vi "Calibrator.vi"(0 "data server address":string="dataserver.cee.cornell.edu", 2 "Channels":T17 items=["SC1Mod1/ai0", "SC1Mod1/ai1", "SC1Mod1/ai2", "SC1Mod1/ai3", "SC1Mod1/ai4", "SC1Mod1/ai5", "SC1Mod1/ai6", "SC1Mod1/ai7", "SC1Mod1/ai8", "SC1Mod1/ai9", "SC1Mod1/ai10", "SC1Mod1/ai11", "SC1Mod1/ai12", "SC1Mod1/ai13", "SC1Mod1/ai14", "SC1Mod1/ai15", "SC1Mod1/ai16", "SC1Mod1/ai17", "SC1Mod1/ai18", "SC1Mod1/ai19", "SC1Mod1/ai20", "SC1Mod1/ai21", "SC1Mod1/ai22", "SC1Mod1/ai23", "SC1Mod1/ai24", "SC1Mod1/ai25", "SC1Mod1/ai26", "SC1Mod1/ai27", "SC1Mod1/ai28", "SC1Mod1/ai29", "SC1Mod1/ai30", "SC1Mod1/ai31", "SC1Mod2/ai0", "SC1Mod2/ai1", "SC1Mod2/ai2", "SC1Mod2/ai3", "SC1Mod2/ai4", "SC1Mod2/ai5", "SC1Mod2/ai6", "SC1Mod2/ai7", "SC1Mod2/ai8", "SC1Mod2/ai9", "SC1Mod2/ai10", "SC1Mod2/ai11", "SC1Mod2/ai12", "SC1Mod2/ai13", "SC1Mod2/ai14", "SC1Mod2/ai15", "SC1Mod2/ai16", "SC1Mod2/ai17", "SC1Mod2/ai18", "SC1Mod2/ai19", "SC1Mod2/ai20", "SC1Mod2/ai21", "SC1Mod2/ai22", "SC1Mod2/ai23", "SC1Mod2/ai24", "SC1Mod2/ai25", "SC1Mod2/ai26", "SC1Mod2/ai27", "SC1Mod2/ai28", "SC1Mod2/ai29", "SC1Mod2/ai30", "SC1Mod2/ai31", "SC1Mod3/ai0", "SC1Mod3/ai1", "SC1Mod3/ai2", "SC1Mod3/ai3", "SC1Mod3/ai4", "SC1Mod3/ai5", "SC1Mod3/ai6", "SC1Mod3/ai7", "SC1Mod3/ai8", "SC1Mod3/ai9", "SC1Mod3/ai10", "SC1Mod3/ai11", "SC1Mod3/ai12", "SC1Mod3/ai13", "SC1Mod3/ai14", "SC1Mod3/ai15", "SC1Mod3/ai16", "SC1Mod3/ai17", "SC1Mod3/ai18", "SC1Mod3/ai19", "SC1Mod3/ai20", "SC1Mod3/ai21", "SC1Mod3/ai22", "SC1Mod3/ai23", "SC1Mod3/ai24", "SC1Mod3/ai25", "SC1Mod3/ai26", "SC1Mod3/ai27", "SC1Mod3/ai28", "SC1Mod3/ai29", "SC1Mod3/ai30", "SC1Mod3/ai31", "SC1Mod4/ai0", "SC1Mod4/ai1", "SC1Mod4/ai2", "SC1Mod4/ai3", "SC1Mod4/ai4", "SC1Mod4/ai5", "SC1Mod4/ai6", "SC1Mod4/ai7", "SC1Mod4/ai8", "SC1Mod4/ai9", "SC1Mod4/ai10", "SC1Mod4/ai11", "SC1Mod4/ai12", "SC1Mod4/ai13", "SC1Mod4/ai14", "SC1Mod4/ai15", "SC1Mod4/ai16", "SC1Mod4/ai17", "SC1Mod4/ai18", "SC1Mod4/ai19", "SC1Mod4/ai20", "SC1Mod4/ai21", "SC1Mod4/ai22", "SC1Mod4/ai23", "SC1Mod4/ai24", "SC1Mod4/ai25", "SC1Mod4/ai26", "SC1Mod4/ai27", "SC1Mod4/ai28", "SC1Mod4/ai29", "SC1Mod4/ai30", "SC1Mod4/ai31"]) -> (7 "sensor file path":path, 9 "Ports out":T17, 10 "Sensor Names":string[](array[string]))   [LabVIEW 2012]
uses:
  toolbar icons/Save configuration.ctl
  toolbar icons/Save calibration.ctl
  toolbar icons/open configuration.ctl
  toolbar icons/Open calibration.ctl
  toolbar icons/simultaneous standard cal.ctl
  toolbar icons/NF90 cal.ctl
  toolbar icons/pH cal.ctl
  toolbar icons/D.O. cal.ctl
  TCP DAQ/Set.ctl
  TCP DAQ/clear offset.ctl
  toolbar icons/Edit calibration.ctl
  toolbar icons/copy sensor.ctl
  toolbar icons/insert sensor.ctl
  toolbar icons/delete sensor.ctl
  DAQ configuration/Sensor array.ctl
  DAQ configuration/channel identifier.ctl
  calibrator graph.ctl
  toolbar icons/help.ctl
  TCP DAQ/Sensor data.ctl
  DAQ configuration/sensor cluster.ctl
  conversion.ctl
  DAQ configuration/scale type.ctl
  correspondence table.ctl
  pH/pH scale.ctl
  Dissolved Oxygen/DO scale.ctl
  calib array.ctl
  TCP DAQ/zero.ctl
  DAQ configuration/Sensor buffer command.ctl
  global scale array.vi
  DataServer/Server Stats.vi
panel:
  out "number of available channels":u16
  in  "Zero":T1
  in  "Sensor List":i32(listbox)=-1
  in  "Save configuration":T2
  in  "Save calibration":T3
  in  "Open configuration":T4
  in  "Open calibration":T5
  in  "units":string
  in  "name":string
  in  "Simultaneous Standard":T6
  in  "nf90":T7
  in  "pH":T8
  in  "DO":T9
  in  "Set clear":T12 {"target value" format="%.1p"}
  in  "Edit calibration":T13
  in  "Cancel":bool
  in  "Duplicate Sensor":T14
  in  "Add Sensor":T15
  in  "Delete Sensor":T16
  in  "OK":bool
  in  "data rate (ms)":u32=10
  in  "history length":u16=100 min=1
  out "Data Display":T19 {"average data rate (Hz)" format="%.2f"; "Min Range" format="%.3f"; "Max Range" format="%.3f"; "Mean (Volts)" format="%.5f"; "Mean (scaled)" format="%.2f"}
  out "Initial Calibration matrix":T20 {"D.O."."K" format="%.6f"; "D.O."."Temperature" format="%.2f"; "pH scale"."Buffers"."V/T" format="%.5f"; "pH scale"."Buffers"."Buffer" format="%.2f"; "pH scale"."Temperature" format="%.2f"; "offset (physical units)" format="%.5f"; "correspondence table"."volts" format="%.4f"; "correspondence table"."physical units" format="%.4f"; "second channel" min=-1; "offset (volts)" format="%.5f"; "conversion matrix" format="%.4e"}
  in  "Volts":T21={"conversion matrix"=[[0.0, 0.0], [0.0, 0.0], [0.0, 0.0], [0.0, 0.0], [0.0, 0.0], [0.0, 0.0]], "units"="volts", "name"="", "scale type"=enum."Volts", "offset (volts)"=0.0, "second channel"=0, "correspondence table"=[], "offset (physical units)"=0.0, "pH scale"={"Buffers"=[], "Temperature"=0.0}, "D.O."={"Temperature"=0.0, "K"=0.0, "barometric pressure"=0.0}} {"D.O."."K" format="%.6f"; "D.O."."Temperature" format="%.2f"; "pH scale"."Buffers"."V/T" format="%.5f"; "pH scale"."Buffers"."Buffer" format="%.2f"; "pH scale"."Temperature" format="%.2f"; "offset (physical units)" format="%.5f"; "correspondence table"."volts" format="%.4f"; "correspondence table"."physical units" format="%.4f"; "second channel" min=-1; "offset (volts)" format="%.5f"; "conversion matrix" format="%.4e"}
  out "Initial Ports":T17
  out "Sensor Data":T26 {"Sensor array"."scaled" format="%.2f"; "Sensor array"."voltage" format="%.4f"; "Time" format="%<%I:%M:%S%2u %p\n%m/%d/%Y>T"}
  in  "Help":T28
  in  "stop":bool
  # "V"
  # "V"
  # "C"
  # "kPa"
  # "C"
  # "C"
  # "kPa"
  # "C"
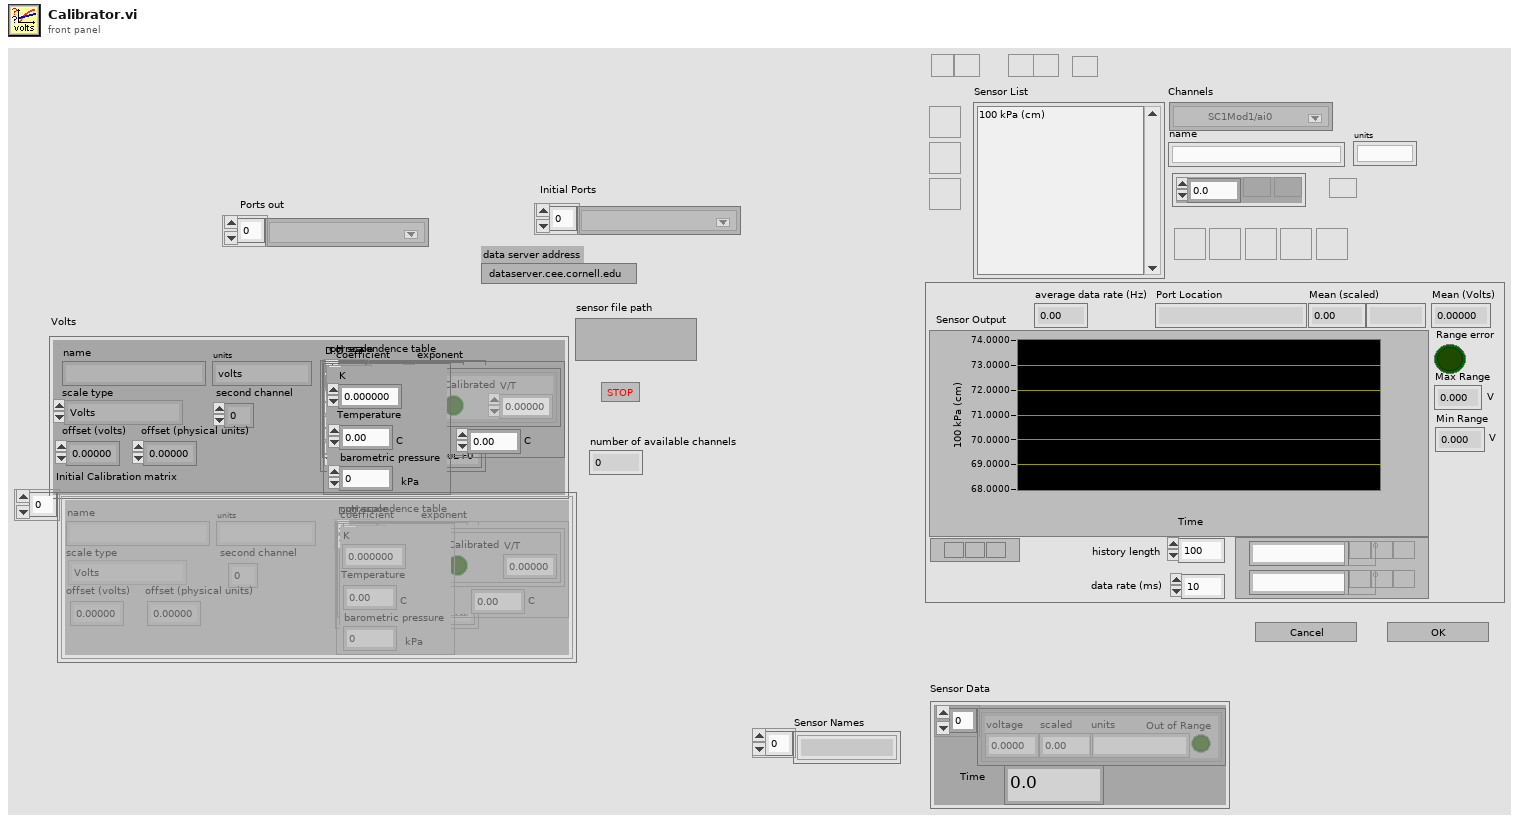
[diagram p1: front panel]
types:
  T1 = typedef "zero.ctl" = bool
  T2 = typedef "Save configuration.ctl" = bool
  T3 = typedef "Save calibration.ctl" = bool
  T4 = typedef "open configuration.ctl" = bool
  T5 = typedef "Open calibration.ctl" = bool
  T6 = typedef "simultaneous standard cal.ctl" = bool
  T7 = typedef "NF90 cal.ctl" = bool
  T8 = typedef "pH cal.ctl" = bool
  T9 = typedef "D.O. cal.ctl" = bool
  T10 = typedef "Set.ctl" = bool
  T11 = typedef "clear offset.ctl" = bool
  T12 = cluster{"Set":T10, "target value":dbl, "Clear":T11}
  T13 = typedef "Edit calibration.ctl" = bool
  T14 = typedef "copy sensor.ctl" = bool
  T15 = typedef "insert sensor.ctl" = bool
  T16 = typedef "delete sensor.ctl" = bool
  T17 = typedef "Sensor array.ctl" = T18[]
  T18 = typedef "channel identifier.ctl" = u16
  T19 = typedef "calibrator graph.ctl" = cluster{"Range error":bool, "Mean (scaled)":dbl, "Mean (Volts)":dbl, "Max Range":dbl, "Min Range":dbl, "units":string, "Sensor Output":cluster{dbl[], dbl[]}[], "Port Location":string, "average data rate (Hz)":dbl}
  T20 = typedef "calib array.ctl" = T21[]
  T21 = typedef "conversion.ctl" = cluster{"conversion matrix":sgl[][], "units":string, "name":string, "scale type":T22, "offset (volts)":dbl, "second channel":i8, "correspondence table":T23, "offset (physical units)":dbl, "pH scale":T24, "D.O.":T25}
  T22 = typedef "scale type.ctl" = enum16{"Volts", "Polynomial", "Correspondence Table", "pH", "Dissolved Oxygen", "Quadratic"}
  T23 = typedef "correspondence table.ctl" = cluster{"physical units":dbl, "volts":dbl}[]
  T24 = typedef "pH scale.ctl" = cluster{"Buffers":cluster{"Buffer":dbl, "Calibrated":bool, "V/T":dbl}[], "Temperature":dbl}
  T25 = typedef "DO scale.ctl" = cluster{"Temperature":dbl, "K":dbl, "barometric pressure":dbl}
  T26 = typedef "Sensor data.ctl" = cluster{" Sensor array":T27[], "Time":dbl}
  T27 = typedef "sensor cluster.ctl" = cluster{"voltage":sgl, "scaled":sgl, "units":string, "Out of Range":bool}
  T28 = typedef "help.ctl" = bool
  T29 = typedef "Sensor buffer command.ctl" = enum16{"read average", "read recent", "read all", "write", "configure", "clear"}
  T30 = typedef "Server stats.ctl" = cluster{"scan rate":dbl, "# connections":i32, "channel settings":cluster{"Name":string, "upper input limits":sgl, "lower input limits":sgl, "Location":string}[]}
  T31 = cluster{"Name":string, "upper input limits":sgl, "lower input limits":sgl, "Location":string}[]
  T32 = cluster{"Name":string, "upper input limits":sgl, "lower input limits":sgl, "Location":string}
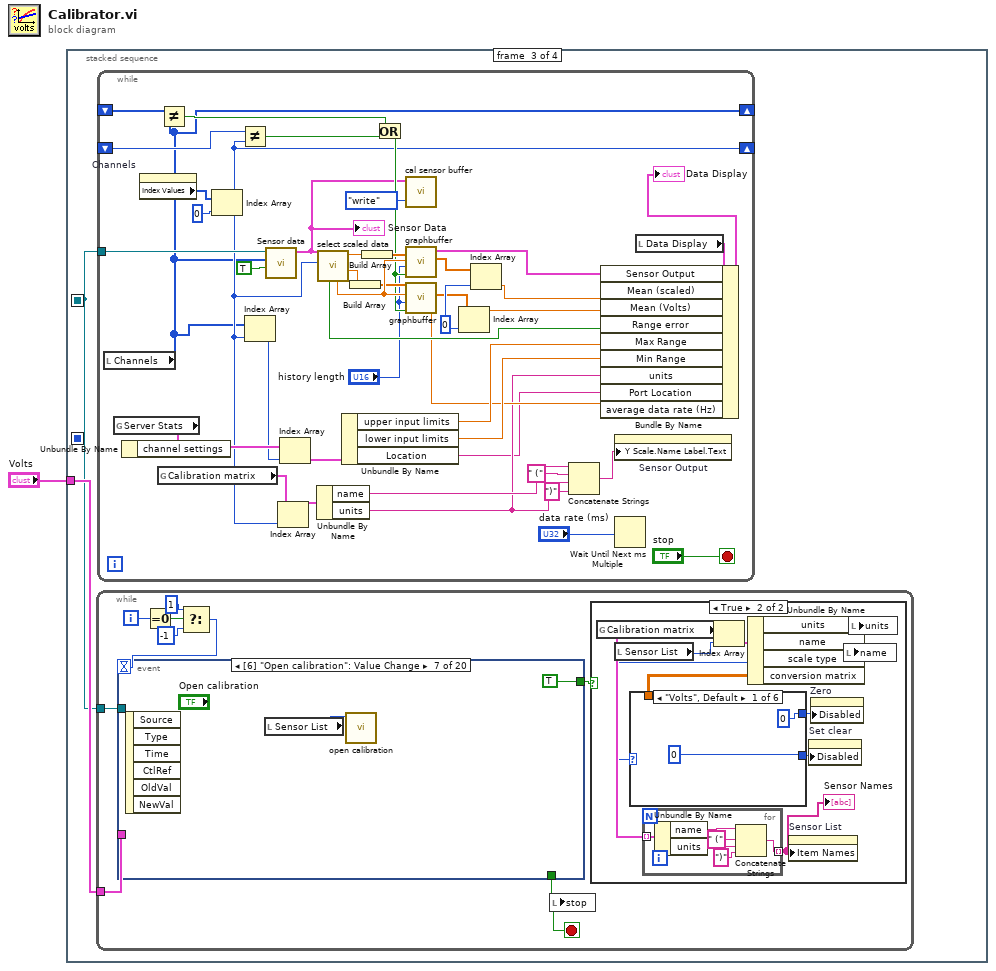
[diagram p0: block diagram]
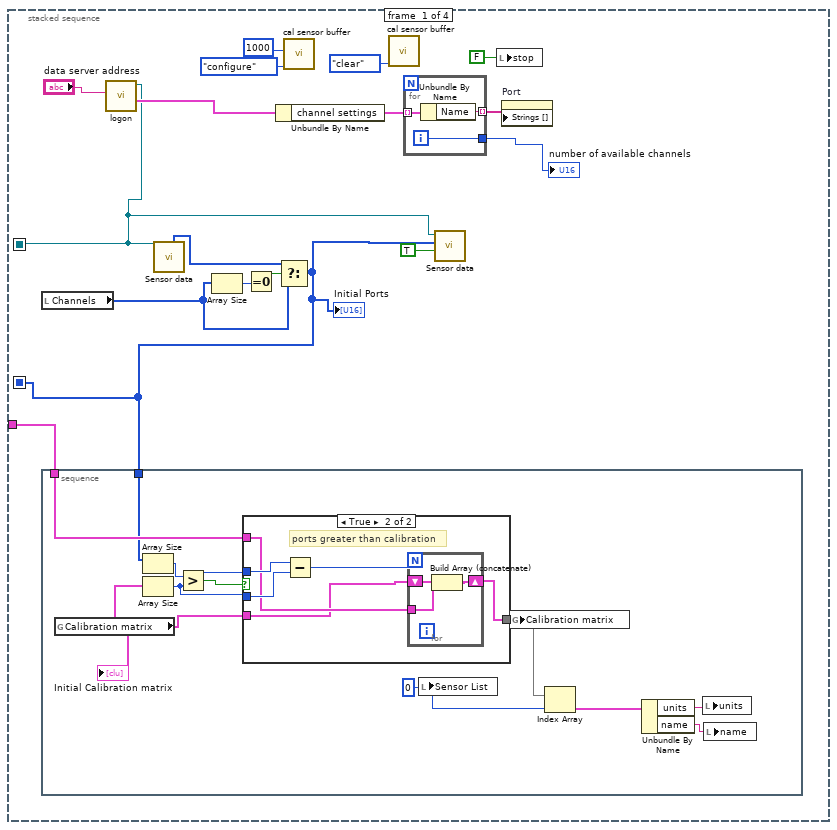
[diagram p2: hidden frame]
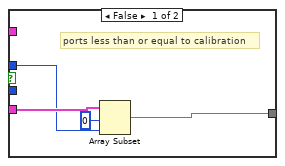
[diagram p3: hidden frame]
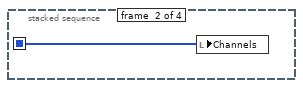
[diagram p4: hidden frame]
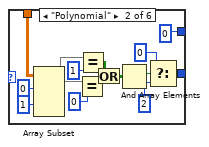
[diagram p6: hidden frame]
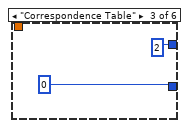
[diagram p7: hidden frame]
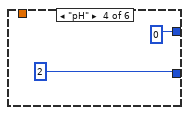
[diagram p8: hidden frame]
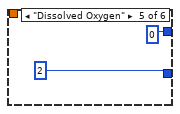
[diagram p9: hidden frame]
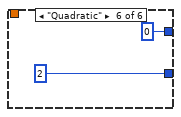
[diagram p10: hidden frame]
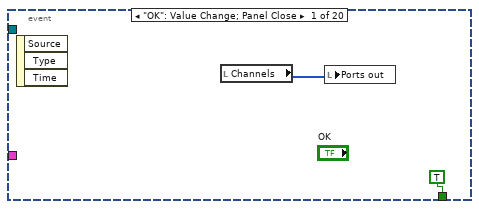
[diagram p11: hidden frame]
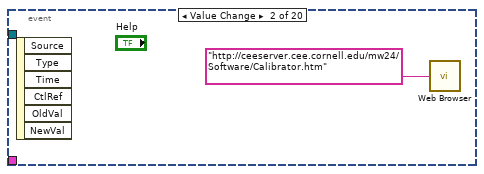
[diagram p12: hidden frame]
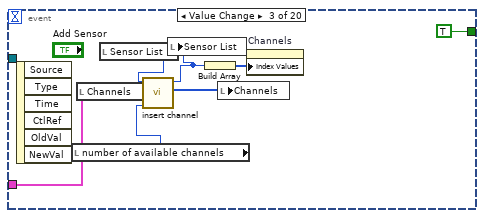
[diagram p13: hidden frame]
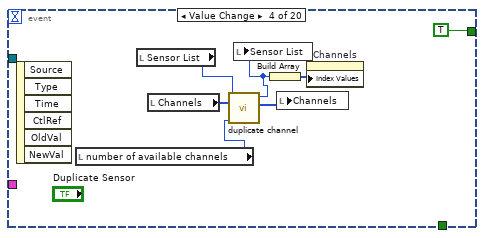
[diagram p14: hidden frame]
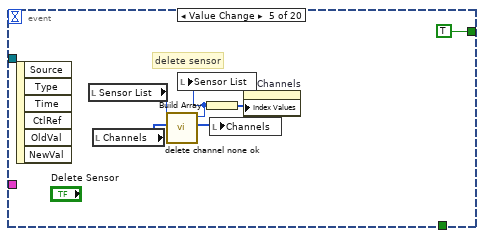
[diagram p15: hidden frame]
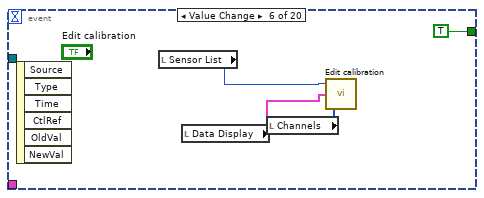
[diagram p16: hidden frame]
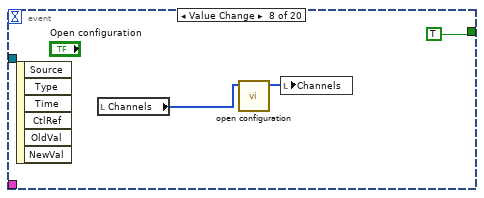
[diagram p17: hidden frame]
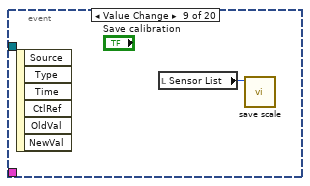
[diagram p18: hidden frame]
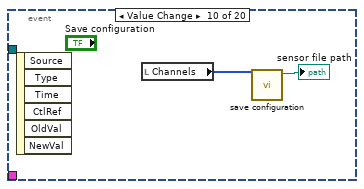
[diagram p19: hidden frame]
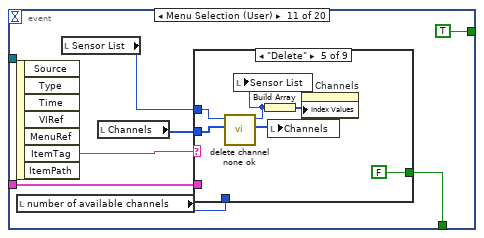
[diagram p20: hidden frame]
diagram:
  n1 = stacked-sequence {
    seq-local: [w6 _ _ _] -> [_ _ w47 w266]
    seq-local: [w2 _ _ _] -> [_ w46 _ _]
    tunnel: "Volts" -> [w18 _ w48 _]
    frame #0 {
      n2 = local read "Channels"() -> (w3:T17)
      n3 = call "logon.vi"("data server address in"="data server address") -> ("Server stats"=w9:T30, "connection ID"=w6:refnum<k5>)  [unwired: 7 in, 2 out]
      n4 = call "Sensor data.vi"("Connection ID in"=w6) -> ("Sensor Array out"=w12:T17)  [unwired: 3 in, 7 out]
      n5 = Array Size(array=w3) -> (size(s)=w11:i32)
      n6 = Equal To 0?(x=w11) -> (x = 0?=w10:bool)
      n7 = Unbundle By Name(w9) -> ("channel settings"=w8:T31)
      n8 = Select(t=w12, s=w10, f=w3) -> (s? t:f=w2:T17)
      "Initial Ports" <- w2
      n9 = stacked-sequence {
        tunnel: w18 -> [w28]
        tunnel: w2 -> [w22]
        frame #0 {
          w27 = u32 0 ("Index")
          n10 = global read "global scale array.vi" "Calibration matrix"() -> (w32:T20)
          "Initial Calibration matrix" <- w32
          n11 = Array Size(array=w22) -> (size(s)=w31:i32)
          n12 = Array Size(array=w32) -> (size(s)=w30:i32)
          n13 = Greater?(x=w31, y=w30) -> (0:w29:bool)
          n14 = case shown="True" w29 {
            tunnel: w31 -> [w35 w42]
            tunnel: w30 -> [_ w41]
            tunnel: w28 -> [_ w40]
            tunnel: w32 -> [w36 w37]
            tunnel: [w33 w38] -> w23
            frame False {
              # "ports less than or equal to calibration"
              n15 = Array Subset(array=w36, index=0 ("Array Index"), length=w35) -> (w33:T20)
            }
            frame True {
              # "ports greater than calibration"
              n16 = Subtract(x=w42, y=w41) -> (x-y=w39:i32)
              n17 = for {
                N: w39 -> [_]
                tunnel: w40 -> [w45]
                shift-right: [w43] -> w38
                shift-left: w37 -> [w44]
                n18 = Build Array (concatenate)(w44, w45) -> (w43:T20)
              }
            }
          }
          n19 = local write "Sensor List"(w27) -> ()
          n20 = global write "global scale array.vi" "Calibration matrix"(w23) -> ()
          n21 = Index Array(array=w23, index=w27) -> (element=w26:T21)
          n22 = Unbundle By Name(w26) -> ("units"=w25:string, "name"=w24:string)
          n23 = local write "units"(w25) -> ()
          n24 = local write "name"(w24) -> ()
        }
      }
      n25 = call "cal sensor buffer.vi"("command"=Sensor_buffer_command."configure", "max array size"=u16 1000) -> ()  [unwired: 3 in, 3 out]
      n26 = call "cal sensor buffer.vi"("command"=Sensor_buffer_command."clear") -> ()  [unwired: 4 in, 3 out]
      n27 = for {
        tunnel: w8 -> [w21] mode=indexing
        tunnel: [w20] -> w7 mode=indexing
        tunnel: [w19] -> w4
        i -> [w19]
        n28 = Unbundle By Name(w21) -> ("Name"=w20:string)
      }
      "number of available channels" <- w4
      n29 = call "Sensor data.vi"("Update channels"=TRUE, "Sensor Array"=w2, "Connection ID in"=w6) -> ()  [unwired: 1 in, 8 out]
      n30 = local write "stop"(FALSE ("stop")) -> ()
      n31 = property on="Port" class="Ring (strict)"("Strings []"=w7) -> ()  [unwired: 2 in, 2 out]
    }
    frame #1 {
      n32 = local write "Channels"(w46) -> ()
    }
    frame #2 {
      n33 = while {
        tunnel: w48 -> [w102]
        tunnel: w47 -> [w95]
        i -> [w100]
        stop <- w94 stop-if-true
        n34 = Equal To 0?(x=w100) -> (x = 0?=w99:bool)
        n35 = Select(t=1, s=w99, f=-1) -> (s? t:f=w96:i32)
        n36 = event shown="[6] \"Open calibration\": Value Change" {
          selector: _ -> [_ _ _ _ _ _ _ _ _ _ _ _ _ _ _ _ _ _ _ _]
          dyn-events: _ -> [_ _ _ _ _ _ _ _ _ _ _ _ _ _ _ _ _ _ _ _]
          timeout: w96 -> [_ _ _ _ _ _ _ _ _ _ _ _ _ _ _ _ _ _ _ _]
          tunnel: [TRUE ("Cancel") _ _ _ _ _ _ _ _ _ w184 _ FALSE ("Cancel") _ _ _ _ _ "Cancel" _] -> w94
          tunnel: w102 -> [_ _ w152 _ _ _ _ _ _ _ w183 _ _ _ _ _ _ _ _ _]
          tunnel: [_ _ TRUE TRUE TRUE TRUE TRUE TRUE _ _ TRUE _ TRUE TRUE TRUE TRUE TRUE TRUE TRUE _] -> w101
          tunnel: w95 -> [_ _ _ _ _ _ _ _ _ _ _ _ _ _ _ _ _ _ w257 _]
          event "OK": Value Change; Panel Close {
            n37 = event-data() -> ()  [unwired: 1 in, 3 out]
            n38 = local read "Channels"() -> (w144:T17)
            n39 = local write "Ports out"(w144) -> ()
          }
          event Value Change {
            n40 = event-data() -> ()  [unwired: 1 in, 6 out]
            n41 = call "Web Browser.vi"("URL"="http://ceeserver.cee.cornell.edu/mw24/Software/Calibrator.htm") -> ()  [unwired: 1 in]
          }
          event Value Change {
            n42 = event-data() -> ()  [unwired: 1 in, 6 out]
            n43 = local read "number of available channels"() -> (w146:u16)
            n44 = local read "Channels"() -> (w149:T17)
            n45 = local read "Sensor List"() -> (w150:i32)
            n46 = call "insert channel.vi"("number of available channels"=w146, "Volts"=w152, "Sensor Array"=w149, "Index"=w150) -> ("Sensor Array out"=w153:T17, "Index out"=w151:u32)  [unwired: 6 in]
            n47 = local write "Sensor List"(w151) -> ()
            n48 = Build Array(w151) -> (w148:u32[])
            n49 = local write "Channels"(w153) -> ()
            n50 = property on="Channels" class="Arr (strict)"("Index Values"=w148) -> ()  [unwired: 2 in, 2 out]
          }
          event Value Change {
            n51 = event-data() -> ()  [unwired: 1 in, 6 out]
            n52 = local read "number of available channels"() -> (w154:u16)
            n53 = local read "Sensor List"() -> (w158:i32)
            n54 = local read "Channels"() -> (w156:T17)
            n55 = call "duplicate channel.vi"("number of available channels"=w154, "Sensor Array"=w156, "Numeric"=w158) -> ("Sensor Array out"=w159:T17, "IndexVals"=w157:u32)  [unwired: 7 in]
            n56 = local write "Sensor List"(w157) -> ()
            n57 = Build Array(w157) -> (w160:u32[])
            n58 = local write "Channels"(w159) -> ()
            n59 = property on="Channels" class="Arr (strict)"("Index Values"=w160) -> ()  [unwired: 2 in, 2 out]
          }
          event Value Change {
            # "delete sensor"
            n60 = event-data() -> ()  [unwired: 1 in, 6 out]
            n61 = local read "Sensor List"() -> (w163:i32)
            n62 = local read "Channels"() -> (w164:T17)
            n63 = call "delete channel none ok.vi"("Sensor Array"=w164, "Indexvals in"=w163) -> ("Sensor Array out"=w165:T17, "Indexvals out"=w162:u32)  [unwired: 8 in]
            n64 = local write "Sensor List"(w162) -> ()
            n65 = Build Array(w162) -> (w166:u32[])
            n66 = local write "Channels"(w165) -> ()
            n67 = property on="Channels" class="Arr (strict)"("Index Values"=w166) -> ()  [unwired: 2 in, 2 out]
          }
          event Value Change {
            n68 = event-data() -> ()  [unwired: 1 in, 6 out]
            n69 = local read "Sensor List"() -> (w170:i32)
            n70 = local read "Data Display"() -> (w169:T19)
            n71 = local read "Channels"() -> (w168:T17)
            n72 = call "Edit calibration.vi"("Ports"=w168, "Data Display"=w169, "Index"=w170) -> ()  [unwired: 2 in]
          }
          event Value Change {
            n73 = event-data() -> ()  [unwired: 1 in, 6 out]
            n74 = local read "Sensor List"() -> (w172:i32)
            n75 = call "open calibration.vi"("Index"=w172) -> ()  [unwired: 6 in, 1 out]
          }
          event Value Change {
            n76 = event-data() -> ()  [unwired: 1 in, 6 out]
            n77 = local read "Channels"() -> (w175:T17)
            n78 = call "open configuration.vi"("Sensor Array"=w175) -> ("Sensor Array out"=w174:T17)  [unwired: 5 in, 1 out]
            n79 = local write "Channels"(w174) -> ()
          }
          event Value Change {
            n80 = event-data() -> ()  [unwired: 1 in, 6 out]
            n81 = local read "Sensor List"() -> (w176:i32)
            n82 = call "save scale.vi"("Index"=w176) -> ()  [unwired: 6 in, 1 out]
          }
          event Value Change {
            n83 = event-data() -> ()  [unwired: 1 in, 6 out]
            n84 = local read "Channels"() -> (w178:T17)
            n85 = call "save configuration.vi"("Sensor Array"=w178) -> ("sensor file path"=→"sensor file path":path)  [unwired: 5 in, 1 out]
          }
          event Menu Selection (User) {
            n86 = event-data() -> ("ItemTag"=w185:string)  [unwired: 1 in, 6 out]
            n87 = local read "number of available channels"() -> (w179:u16)
            n88 = local read "Sensor List"() -> (w181:i32)
            n89 = local read "Channels"() -> (w182:T17)
            n90 = case shown="\"Delete\"" w185 {
              tunnel: w181 -> [_ _ w192 w201 w207 w213 w216 w218 _]
              tunnel: w182 -> [w187 w188 w194 w200 w206 w211 _ _ w220]
              tunnel: [FALSE TRUE FALSE FALSE FALSE FALSE FALSE FALSE FALSE] -> w184
              tunnel: w183 -> [_ _ w193 _ _ _ _ _ _]
              tunnel: w179 -> [_ _ w190 w198 _ _ _ _ _]
              frame "Save Method", Default {
                n91 = call "save configuration.vi"("Sensor Array"=w187) -> ()  [unwired: 5 in, 2 out]
              }
              frame "Close" {
                n92 = local write "Ports out"(w188) -> ()
              }
              frame "Insert New" {
                n93 = call "insert channel.vi"("number of available channels"=w190, "Volts"=w193, "Sensor Array"=w194, "Index"=w192) -> ("Sensor Array out"=w196:T17, "Index out"=w191:u32)  [unwired: 6 in]
                n94 = local write "Sensor List"(w191) -> ()
                n95 = control-ref of="Sensor List"() -> ()  [unwired: 1 out]
                n96 = Build Array(w191) -> (w195:u32[])
                n97 = local write "Channels"(w196) -> ()
                n98 = property on="Channels" class="Arr (strict)"("Index Values"=w195) -> ()  [unwired: 2 in, 2 out]
              }
              frame "Copy" {
                n99 = call "duplicate channel.vi"("number of available channels"=w198, "Sensor Array"=w200, "Numeric"=w201) -> ("Sensor Array out"=w202:T17, "IndexVals"=w199:u32)  [unwired: 7 in]
                n100 = local write "Sensor List"(w199) -> ()
                n101 = Build Array(w199) -> (w203:u32[])
                n102 = local write "Channels"(w202) -> ()
                n103 = property on="Channels" class="Arr (strict)"("Index Values"=w203) -> ()  [unwired: 2 in, 2 out]
              }
              frame "Delete" {
                n104 = call "delete channel none ok.vi"("Sensor Array"=w206, "Indexvals in"=w207) -> ("Sensor Array out"=w208:T17, "Indexvals out"=w205:u32)  [unwired: 8 in]
                n105 = local write "Sensor List"(w205) -> ()
                n106 = Build Array(w205) -> (w209:u32[])
                n107 = local write "Channels"(w208) -> ()
                n108 = property on="Channels" class="Arr (strict)"("Index Values"=w209) -> ()  [unwired: 2 in, 2 out]
              }
              frame "Edit" {
                n109 = local read "Data Display"() -> (w212:T19)
                n110 = call "Edit calibration.vi"("Ports"=w211, "Data Display"=w212, "Index"=w213) -> ()  [unwired: 2 in]
              }
              frame "Save" {
                n111 = call "save scale.vi"("Index"=w216) -> ()  [unwired: 6 in, 1 out]
              }
              frame "Open" {
                n112 = call "open calibration.vi"("Index"=w218) -> ()  [unwired: 6 in, 1 out]
              }
              frame "Open Method" {
                n113 = call "open configuration.vi"("Sensor Array"=w220) -> ("Sensor Array out"=w221:T17)  [unwired: 5 in, 1 out]
                n114 = local write "Channels"(w221) -> ()
              }
            }
          }
          event "Set clear": Value Change {
            n115 = event-data() -> ()  [unwired: 1 in, 6 out]
            n116 = local read "Sensor List"() -> (w222:i32)
            n117 = call "Set or Clear value.vi"("Set clear"="Set clear", "Index"=w222) -> ()  [unwired: 2 in]
          }
          event "Sensor List": Value Change; Timeout {
            n118 = event-data() -> ()  [unwired: 1 in, 3 out]
            n119 = Array Size(array="Channels") -> (size(s)=w230:i32)
            n120 = Decrement(x=w230) -> (x-1=w228:i32)
            n121 = Greater?(x="Sensor List", y=w228) -> (0:w227:bool)
            n122 = case shown="False" w227 {
              tunnel: [w233 w234] -> w229
              tunnel: "Sensor List" -> [w233 _]
              tunnel: w228 -> [_ w234]
              frame False {
              }
              frame True {
                n123 = local write "Sensor List"(w234) -> ()
              }
            }
            n124 = Build Array(w229) -> (w226:i32[])
            n125 = property on="Channels" class="Arr (strict)"("Index Values"=w226) -> ()  [unwired: 2 in, 2 out]
          }
          event "units", "name": Value Change {
            n126 = event-data() -> ()  [unwired: 1 in, 6 out]
            n127 = local read "Sensor List"() -> (w240:i32)
            n128 = global read "global scale array.vi" "Calibration matrix"() -> (w241:T20)
            n129 = Index Array(array=w241, index=w240) -> (element=w239:T21)
            n130 = Bundle By Name(cluster=w239, "units"="units", "name"="name") -> (w238:T21)
            n131 = Replace Array Subset(array=w241, new element=w238, index=w240) -> (w242:T20)
            n132 = global write "global scale array.vi" "Calibration matrix"(w242) -> ()
          }
          event Value Change {
            n133 = event-data() -> ()  [unwired: 1 in, 6 out]
            n134 = local read "Sensor List"() -> (w244:i32)
            n135 = call "calibrate DO.vi"("Index"=w244) -> ()  [unwired: 11 in]
          }
          event Value Change {
            n136 = event-data() -> ()  [unwired: 1 in, 6 out]
            n137 = local read "Sensor List"() -> (w245:i32)
            n138 = call "pH calibration.vi"("pH index"=w245) -> ()  [unwired: 11 in]
          }
          event Value Change {
            n139 = event-data() -> ()  [unwired: 1 in, 6 out]
            n140 = local read "data server address"() -> (w247:string)
            n141 = local read "Sensor List"() -> (w249:i32)
            n142 = local read "Channels"() -> (w250:T17)
            n143 = call "NF90 calibrator.vi"("Ports"=w250, "channel index"=w249, "data server address"=w247) -> ()  [unwired: 9 in]
          }
          event Value Change {
            n144 = event-data() -> ()  [unwired: 1 in, 6 out]
            n145 = local read "data server address"() -> (w253:string)
            n146 = local read "Channels"() -> (w251:T17)
            n147 = local read "Sensor List"() -> (w252:i32)
            n148 = call "Simultaneous Standard.vi"("data server address"=w253, "Uncalibrated Index"=w252, "Ports"=w251) -> ()  [unwired: 5 in]
          }
          event "Cancel": Value Change {
            n149 = event-data() -> ()  [unwired: 1 in, 6 out]
            n150 = local read "Initial Calibration matrix"() -> (w259:T20)
            n151 = local read "Initial Ports"() -> (w258:T17)
            "Ports out" <- w258
            n152 = global write "global scale array.vi" "Calibration matrix"(w259) -> ()
            n153 = call "Sensor data.vi"("Update channels"=TRUE, "Sensor Array"=w258, "Connection ID in"=w257) -> ()  [unwired: 1 in, 8 out]
          }
          event Value Change {
            n154 = event-data() -> ()  [unwired: 1 in, 6 out]
            n155 = call "cal sensor buffer.vi"("command"=Sensor_buffer_command."read average", "smooth interval (s)"=sgl 5.0) -> ("Sensor Data smoothed"=w264:T26)  [unwired: 3 in, 2 out]
            n156 = local read "Sensor List"() -> (w263:i32)
            n157 = call "select scaled data.vi"("Sensor index"=w263, "Sensor Data"=w264) -> ("voltage"=w262:sgl)  [unwired: 4 in, 5 out]
            n158 = call "zero channel.vi"("Index"=w263, "Mean (Volts)"=w262) -> ()  [unwired: 6 in]
          }
        }
        n159 = local write "stop"(w94) -> ()
        n160 = case shown="True" w101 {
          frame False {
          }
          frame True {
            n161 = global read "global scale array.vi" "Calibration matrix"() -> (w108:T20)
            n162 = local read "Sensor List"() -> (w109:i32)
            n163 = for {
              tunnel: w108 -> [w142] mode=indexing
              tunnel: [w137] -> w104 mode=indexing
              n164 = Unbundle By Name(w142) -> ("name"=w141:string, "units"=w139:string)
              n165 = Concatenate Strings(w141, " (" ("string"), w139, ")" ("string")) -> (w137:string)
            }
            "Sensor Names" <- w104
            n166 = Index Array(array=w108, index=w109) -> (element=w110:T21)
            n167 = Unbundle By Name(w110) -> ("units"=w112:string, "name"=w111:string, "scale type"=w107:T22, "conversion matrix"=w105:sgl[][])
            n168 = case shown="\"Volts\", Default" w107 {
              tunnel: [u8 0 ("Disabled") w116 u8 0 ("Disabled") u8 2 ("Disabled") u8 2 ("Disabled") u8 2 ("Disabled")] -> w106
              tunnel: w105 -> [_ w128 _ _ _ _]
              tunnel: [u8 0 ("Disabled") u8 0 ("Disabled") u8 2 ("Disabled") u8 0 ("Disabled") u8 0 ("Disabled") u8 0 ("Disabled")] -> w103
              frame "Volts", Default {
              }
              frame "Polynomial" {
                n169 = Array Subset(array=w128, index (row)=0 ("index"), index (col)=1 ("index")) -> (w123:sgl[][])  [unwired: 2 in]
                n170 = Equal?(x=w123, y=u8 0 ("Disabled")) -> (x = y?=w121:bool[][])
                n171 = Equal?(x=w123, y=u8 1 ("Disabled")) -> (x = y?=w122:bool[][])
                n172 = Or(x=w122, y=w121) -> (x .or. y?=w120:bool[][])
                n173 = And Array Elements(Boolean array=w120) -> (logical AND=w118:bool)
                n174 = Select(t=u8 0 ("Disabled"), s=w118, f=u8 2 ("Disabled")) -> (s? t:f=w116:u8)
              }
              frame "Correspondence Table" {
              }
              frame "pH" {
              }
              frame "Dissolved Oxygen" {
              }
              frame "Quadratic" {
              }
            }
            n175 = property on="Sensor List" class="LstBox (strict)"("Item Names"=w104) -> ()  [unwired: 2 in, 2 out]
            n176 = property on="Set clear" class="Clust"("Disabled"=w106) -> ()  [unwired: 2 in, 2 out]
            n177 = property on="Zero" class="Bool"("Disabled"=w103) -> ()  [unwired: 2 in, 2 out]
            n178 = local write "name"(w111) -> ()
            n179 = local write "units"(w112) -> ()
          }
        }
      }
      n180 = while {
        shift-left: _ -> [w83]
        shift-right: [w52] -> _
        shift-left: _ -> [w84]
        shift-right: [w49] -> _
        tunnel: w47 -> [w63]
        stop <- "stop" stop-if-true
        w91 = 0 ("Index")
        n181 = local read "Channels"() -> (w49:T17)
        n182 = global read "Server Stats.vi" "Server Stats"() -> (w56:T30)
        n183 = Unbundle By Name(w56) -> ("channel settings"=w55:T31)
        n184 = property on="Channels" class="Arr (strict)"() -> ("Index Values"=w66:u32[])  [unwired: 2 in, 2 out]
        n185 = global read "global scale array.vi" "Calibration matrix"() -> (w57:T20)
        n186 = Not Equal?(x=w84, y=w49) -> (x != y?=w82:bool)
        n187 = Index Array(array=w66, index=0 ("Index")) -> (element=w52:u32)
        n188 = Not Equal?(x=w83, y=w52) -> (x != y?=w81:bool)
        n189 = Index Array(array=w49, index=w52) -> (element=w51:T18)
        n190 = call "Sensor data.vi"("Update channels"=TRUE, "Sensor Array"=w49, "Connection ID in"=w63) -> ("Sensor Data"=w64:T26)  [unwired: 1 in, 7 out]
        "Sensor Data" <- w64
        n191 = Index Array(array=w57, index=w52) -> (element=w80:T21)
        n192 = Index Array(array=w55, index=w51) -> (element=w54:T32)
        n193 = Unbundle By Name(w80) -> ("name"=w62:string, "units"=w60:string)
        n194 = call "select scaled data.vi"("Sensor index"=w52, "Sensor Data"=w64) -> ("voltage"=w87:sgl, "scaled"=w93:sgl, "Time"=w88:dbl, "Out of Range"=w75:bool)  [unwired: 4 in, 2 out]
        n195 = Unbundle By Name(w54) -> ("upper input limits"=w74:sgl, "lower input limits"=w73:sgl, "Location"=w53:string)
        n196 = Build Array(w87) -> (w86:sgl[])
        n197 = Build Array(w93) -> (w92:sgl[])
        n198 = Or(x=w82, y=w81) -> (x .or. y?=w71:bool)
        n199 = call "cal sensor buffer.vi"("command"=Sensor_buffer_command."write", "Sensor Data"=w64) -> ()  [unwired: 3 in, 3 out]
        n200 = call "graphbuffer.vi"("Reset"=w71, "history length"="history length", "Time"=w88, "data"=w92) -> ("Mean"=w85:dbl[], "Multiplot graph data"=w78:cluster{dbl[], dbl[]}[])  [unwired: 5 in, 1 out]
        n201 = call "graphbuffer.vi"("Reset"=w71, "history length"="history length", "Time"=w88, "data"=w86) -> ("data rate (Hz)"=w72:dbl, "Mean"=w89:dbl[])  [unwired: 5 in, 1 out]
        n202 = Index Array(array=w89, index=w91) -> (element=w76:dbl)
        n203 = Index Array(array=w85, index=w91) -> (element=w77:dbl)
        n204 = Concatenate Strings(w62, " (" ("string"), w60, ")" ("string")) -> (w58:string)
        n205 = property on="Sensor Output" class="XYGraph (strict)"("Y Scale.Name Label.Text"=w58) -> ()  [unwired: 2 in, 2 out]
        n206 = Wait Until Next ms Multiple(millisecond multiple="data rate (ms)") -> ()  [unwired: 1 out]
        n207 = local read "Data Display"() -> (w79:T19)
        n208 = Bundle By Name(cluster=w79, "Sensor Output"=w78, "Mean (scaled)"=w77, "Mean (Volts)"=w76, "Range error"=w75, "Max Range"=w74, "Min Range"=w73, "units"=w60, "Port Location"=w53, "average data rate (Hz)"=w72) -> (→"Data Display":T19)
      }
    }
    frame #3 {
      n209 = call "logoff tcp.vi"("Connection ID"=w266) -> ()  [unwired: 9 in, 2 out]
    }
  }
